vi "ViperHawk Compile Data.vi"(10 "logData in":T1, 11 "Diagnostic in":T2) -> (3 "Diagnostic out":T2)   [LabVIEW 2014]
uses:
  Type Definitions/ViperHawk/ViperHawk Diagnostic Data.ctl
  Type Definitions/ViperHawk/ViperHawk logData.ctl
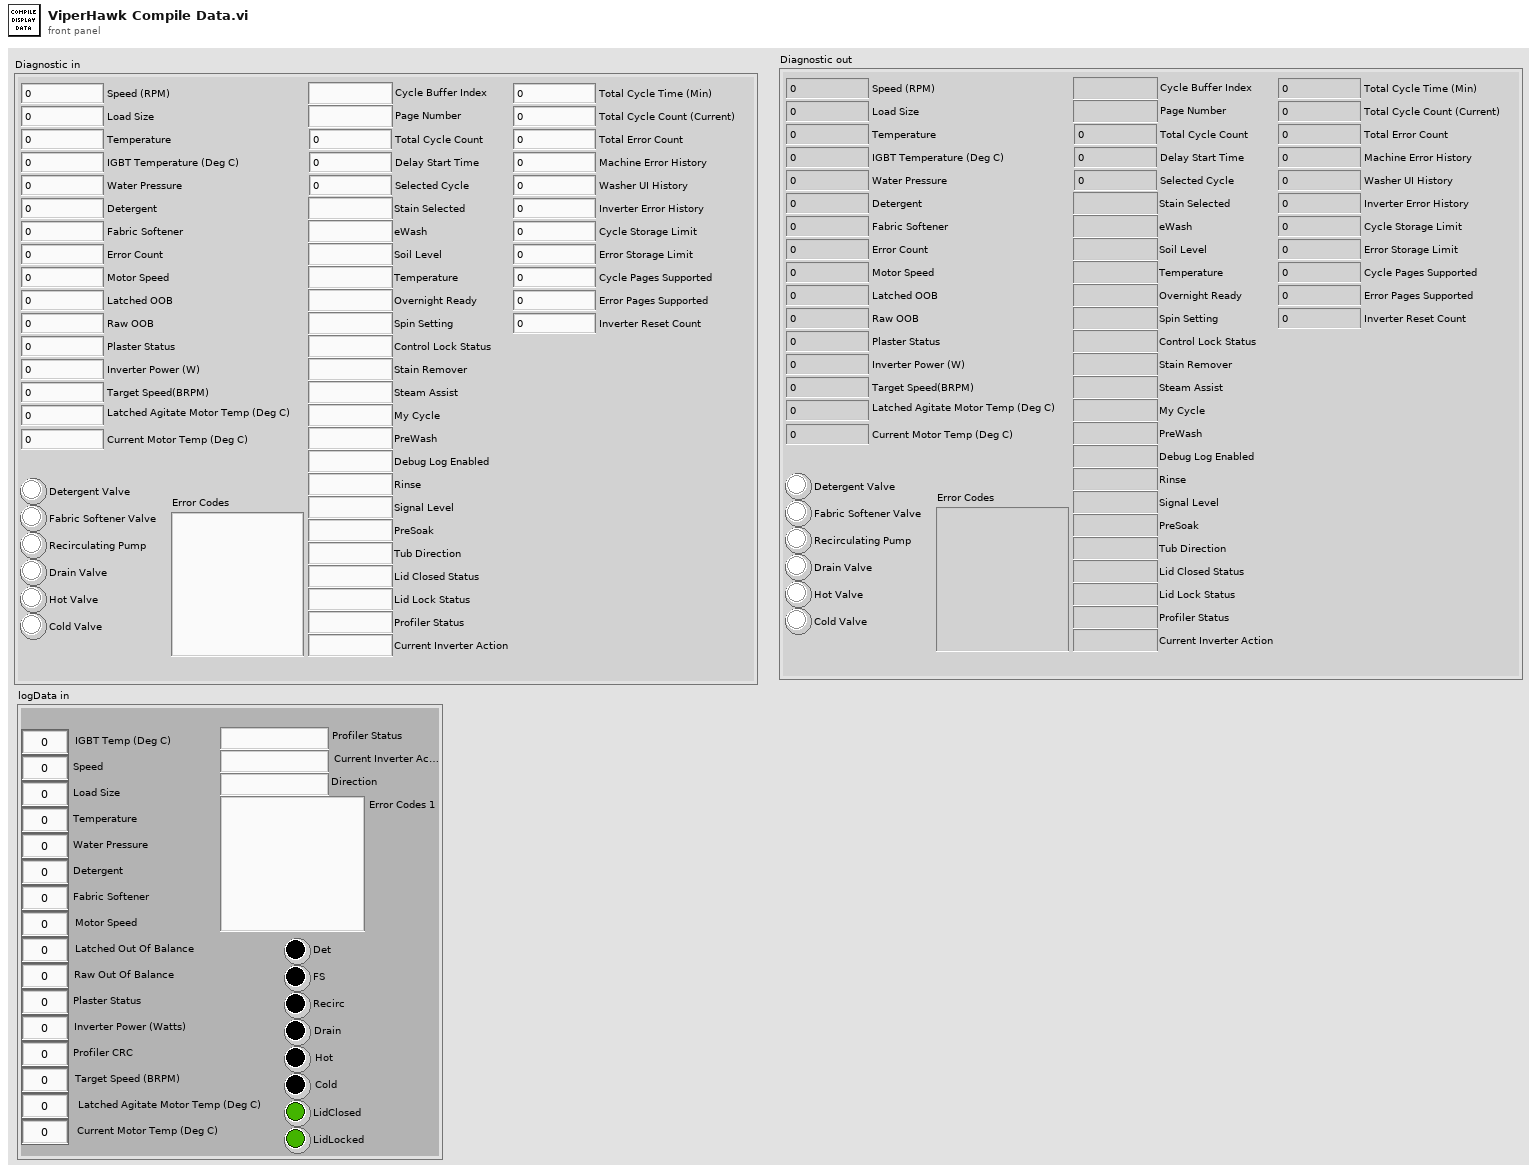
[diagram p1: front panel]
types:
  T1 = typedef "ViperHawk logData.ctl" = cluster{"IGBT Temp (Deg C)":u8, "Speed":u32, "Load Size":u32, "Temperature":u8, "Water Pressure":u32, "Detergent":u32, "Fabric Softener":u32, "Direction":string, "Det":bool, "FS":bool, "Recirc":bool, "Drain":bool, "Hot":bool, "Cold":bool, "LidClosed":bool, "LidLocked":bool, "Motor Speed":u16, "Latched Out Of Balance":u16, "Raw Out Of Balance":u16, "Plaster Status":u8, "Inverter Power (Watts)":u16, "Profiler Status":string, "Profiler CRC":u16, "Current Inverter Action":string, "Target Speed (BRPM)":u16, "Latched Agitate Motor Temp (Deg C)":u8, "Current Motor Temp (Deg C)":u8, "Error Codes 1":string}
  T2 = typedef "ViperHawk Diagnostic Data.ctl" = cluster{"Cycle Buffer Index":string, "Page Number":string, "Total Cycle Count":u32, "Delay Start Time":u32, "Stain Selected":string, "Selected Cycle":u32, "eWash":string, "Soil Level":string, "Temperature":string, "Overnight Ready":string, "Spin Setting":string, "Control Lock Status":string, "Stain Remover":string, "Steam Assist":string, "My Cycle":string, "PreWash":string, "Debug Log Enabled":string, "Rinse":string, "Signal Level":string, "PreSoak":string, "Speed (RPM)":u32, "Load Size":u32, "Temperature":u32, "Water Pressure":u32, "Detergent":u32, "Fabric Softener":u32, "Tub Direction":string, "Detergent Valve":bool, "Fabric Softener Valve":bool, "Recirculating Pump":bool, "Drain Valve":bool, "Hot Valve":bool, "Cold Valve":bool, "Lid Closed Status":string, "Lid Lock Status":string, "Error Count":u32, "IGBT Temperature (Deg C)":u32, "Motor Speed":u32, "Latched OOB":u32, "Raw OOB":u32, "Plaster Status":u32, "Inverter Power (W)":u32, "Target Speed(BRPM)":u32, "Latched Agitate Motor Temp (Deg C)":u32, "Current Motor Temp (Deg C)":u32, "Profiler Status":string, "Current Inverter Action":string, "Error Codes":string, "Total Cycle Time (Min)":u32, "Total Cycle Count (Current)":u16, "Total Error Count":u16, "Machine Error History":u32, "Washer UI History":u32, "Inverter Error History":u32, "Cycle Storage Limit":u8, "Error Storage Limit":u8, "Cycle Pages Supported":u8, "Error Pages Supported":u8, "Inverter Reset Count":u16}
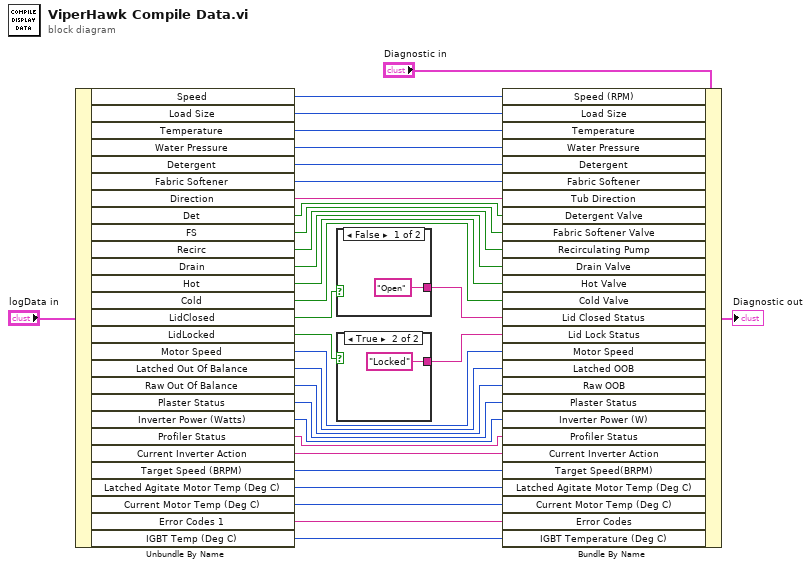
[diagram p0: block diagram]
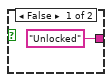
[diagram p2: hidden frame]
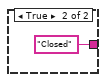
[diagram p3: hidden frame]
diagram:
  n1 = Unbundle By Name("logData in") -> ("Speed"=w25:u32, "Load Size"=w24:u32, "Temperature"=w23:u8, "Water Pressure"=w22:u32, "Detergent"=w21:u32, "Fabric Softener"=w20:u32, "Direction"=w19:string, "Det"=w18:bool, "FS"=w17:bool, "Recirc"=w16:bool, "Drain"=w15:bool, "Hot"=w14:bool, "Cold"=w13:bool, "LidClosed"=w27:bool, "LidLocked"=w26:bool, "Motor Speed"=w12:u16, "Latched Out Of Balance"=w11:u16, "Raw Out Of Balance"=w10:u16, "Plaster Status"=w9:u8, "Inverter Power (Watts)"=w8:u16, "Profiler Status"=w7:string, "Current Inverter Action"=w6:string, "Target Speed (BRPM)"=w5:u16, "Latched Agitate Motor Temp (Deg C)"=w4:u8, "Current Motor Temp (Deg C)"=w3:u8, "Error Codes 1"=w2:string, "IGBT Temp (Deg C)"=w1:u8)
  n2 = case shown="False" w27 {
    tunnel: ["Open" "Closed"] -> w32
    frame False {
    }
    frame True {
    }
  }
  n3 = case shown="True" w26 {
    tunnel: ["Unlocked" "Locked"] -> w31
    frame False {
    }
    frame True {
    }
  }
  n4 = Bundle By Name(cluster="Diagnostic in", "Speed (RPM)"=w25, "Load Size"=w24, "Temperature"=w23, "Water Pressure"=w22, "Detergent"=w21, "Fabric Softener"=w20, "Tub Direction"=w19, "Detergent Valve"=w18, "Fabric Softener Valve"=w17, "Recirculating Pump"=w16, "Drain Valve"=w15, "Hot Valve"=w14, "Cold Valve"=w13, "Lid Closed Status"=w32, "Lid Lock Status"=w31, "Motor Speed"=w12, "Latched OOB"=w11, "Raw OOB"=w10, "Plaster Status"=w9, "Inverter Power (W)"=w8, "Profiler Status"=w7, "Current Inverter Action"=w6, "Target Speed(BRPM)"=w5, "Latched Agitate Motor Temp (Deg C)"=w4, "Current Motor Temp (Deg C)"=w3, "Error Codes"=w2, "IGBT Temperature (Deg C)"=w1) -> (→"Diagnostic out":T2)
